vi "XMLPublishNode.vi"(8 "Error In":errorcluster, 9 "parent opcua path":string, 10 "OPC UA server refnum in":refnum<k21>, 11 "DOM node":refnum<k20>) -> (0 "Error Out":errorcluster, 2 "OPC UA server refnum out":refnum<k21>, 3 "DOM node (dup)":refnum<k20>)   [LabVIEW 2014, in "OPCUA XML.lvlib"]
uses:
  OPCUA XML.lvlib
  <vilib>/xml/Close Reference(Node).vi
  <vilib>/xml/Close Reference(NNMap).vi
  <resource>/objmgr/DOMUserDefRef.rc
  <vilib>/xml/NI_XML.lvlib
  <vilib>/OPCUA/NI OPC UA Server.lvlib
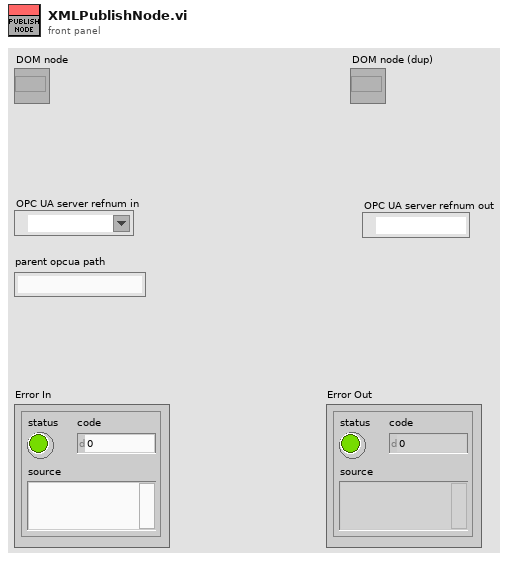
[diagram p1: front panel]
types:
  T1 = cluster{"name":string, "data type":u16, "access level":u16, "description":string}
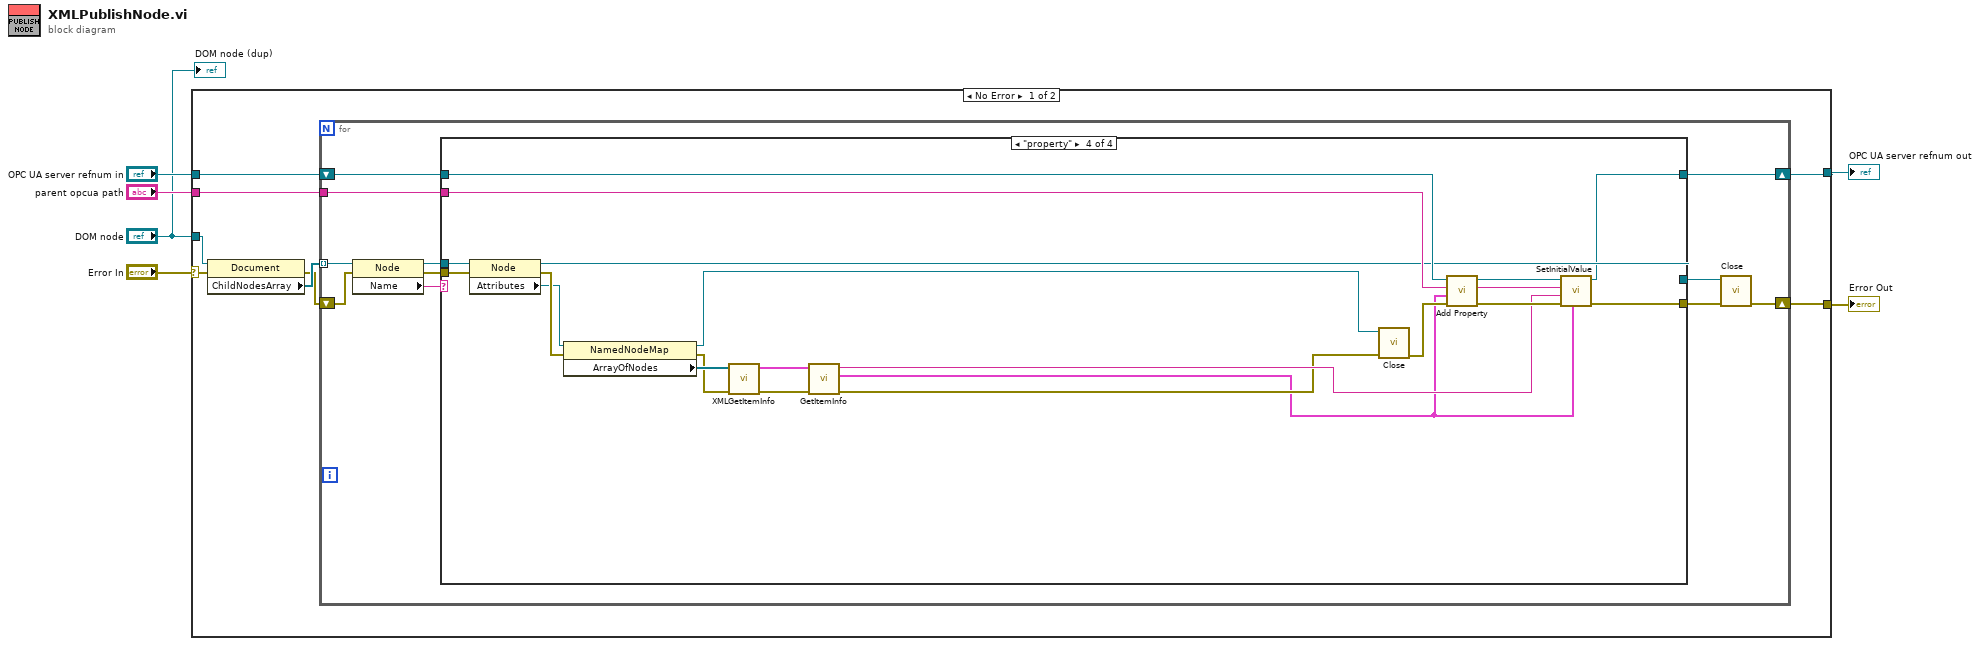
[diagram p0: block diagram]
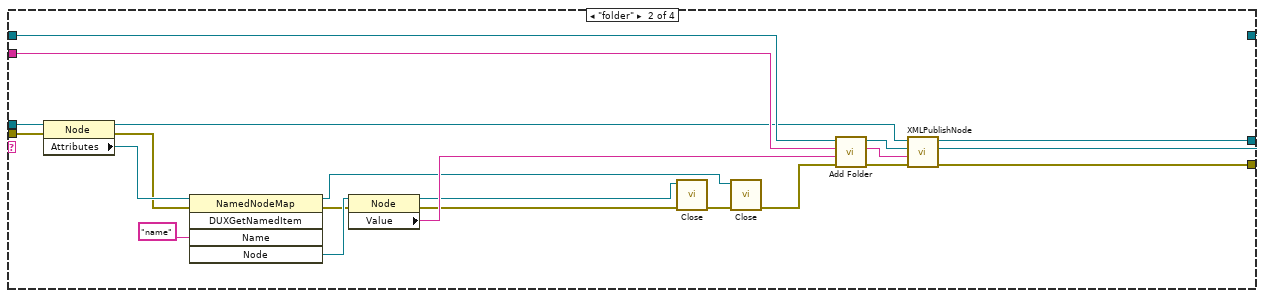
[diagram p3: hidden frame]
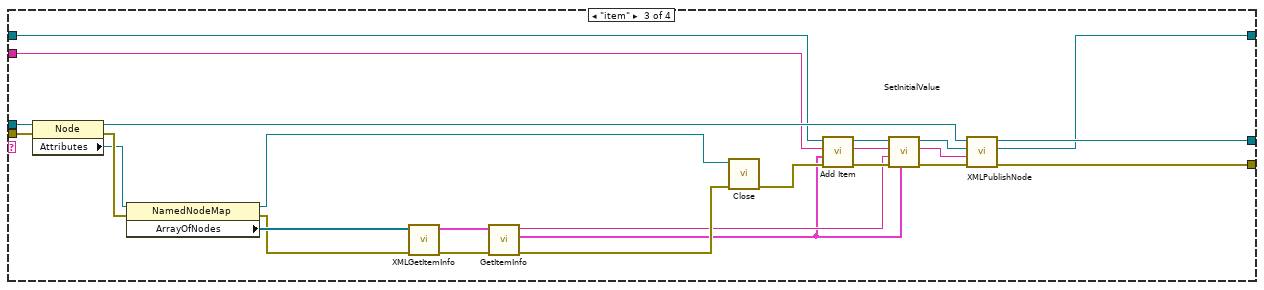
[diagram p4: hidden frame]
diagram:
  n1 = case shown="No Error" "Error In" {
    selector: "Error In" -> [w8 w98]
    tunnel: [w12 w98] -> w6
    tunnel: "DOM node" -> [w14 _]
    tunnel: "parent opcua path" -> [w11 _]
    tunnel: "OPC UA server refnum in" -> [w10 w97]
    tunnel: [w9 w97] -> w2
    frame No Error {
      n2 = property class="Document"(reference=w14, error in=w8) -> (error out=w7:errorcluster, "ChildNodesArray"=w13:refnum<k20>[])  [unwired: 1 out]
      n3 = for {
        tunnel: w13 -> [w25] mode=indexing
        shift-right: [w21] -> w12
        shift-left: w7 -> [w22]
        tunnel: w11 -> [w20]
        shift-right: [w18] -> w9
        shift-left: w10 -> [w19]
        n4 = property class="Node"(reference=w25, error in=w22) -> (reference out=w23:refnum<k20>, error out=w17:errorcluster, "Name"=w24:string)
        n5 = case shown="\"property\"" w24 {
          tunnel: w23 -> [w27 w50 w75 w91]
          tunnel: w20 -> [_ w46 w71 w95]
          tunnel: w19 -> [w26 w45 w72 w96]
          tunnel: [w26 w39 w70 w85] -> w18
          tunnel: w17 -> [w28 w36 w68 w90]
          tunnel: [w27 w42 w74 w89] -> w16
          tunnel: [w28 w41 w69 w84] -> w15
          frame Default {
          }
          frame "folder" {
            n6 = property class="Node"(reference=w50, error in=w36) -> (reference out=w43:refnum<k20>, error out=w35:errorcluster, "Attributes"=w49:refnum<k20>)
            n7 = invoke class="NamedNodeMap" method="DUXGetNamedItem"(reference=w49, error in=w35, "Name"="name") -> (reference out=w30:refnum<k20>, error out=w34:errorcluster, "Node"=w47:refnum<k20>)  [unwired: 2 in, 2 out]
            n8 = property class="Node"(reference=w47, error in=w34) -> (reference out=w29:refnum<k20>, error out=w33:errorcluster, "Value"=w44:string)
            n9 = call-poly <vilib>:"Close.vi"("error in (no error)"=w33, "node"=w29) -> ("error out"=w32:errorcluster)  [unwired: 7 out]
            n10 = call-poly <vilib>:"Close.vi"("error in (no error)"=w32, "named node map"=w30) -> ("error out"=w31:errorcluster)  [unwired: 7 out]
            n11 = call <vilib>:"Add Folder.vi"("error in (no error)"=w31, "folder name"=w44, "parent folder path"=w46, "OPC UA server refnum in"=w45) -> ("error out"=w37:errorcluster, "folder path"=w38:string, "OPC UA server refnum out"=w40:refnum<k21>)  [unwired: 4 in]
            n12 = call "XMLPublishNode.vi"("Error In"=w37, "parent opcua path"=w38, "OPC UA server refnum in"=w40, "DOM node"=w43) -> ("Error Out"=w41:errorcluster, "OPC UA server refnum out"=w39:refnum<k21>, "DOM node (dup)"=w42:refnum<k20>)  [unwired: 5 in]
          }
          frame "item" {
            n13 = property class="Node"(reference=w75, error in=w68) -> (reference out=w73:refnum<k20>, error out=w67:errorcluster, "Attributes"=w66:refnum<k20>)
            n14 = property class="NamedNodeMap"(reference=w66, error in=w67) -> (reference out=w65:refnum<k20>, error out=w56:errorcluster, "ArrayOfNodes"=w57:refnum<k20>[])
            n15 = call "XMLGetItemInfo.vi"("error in (no error)"=w56, "ArrayOfNodes"=w57) -> ("error out"=w55:errorcluster, "Array"=w54:cluster{"Name":string, "Value":string}[])  [unwired: 8 in]
            n16 = call "GetItemInfo.vi"("error in (no error)"=w55, "Array"=w54) -> ("error out"=w53:errorcluster, "item"=w51:T1, "Value"=w52:string)  [unwired: 7 in]
            n17 = call-poly <vilib>:"Close.vi"("error in (no error)"=w53, "named node map"=w65) -> ("error out"=w64:errorcluster)  [unwired: 7 out]
            n18 = call <vilib>:"Add Item.vi"("error in (no error)"=w64, "item"=w51, "parent folder path"=w71, "OPC UA server refnum in"=w72) -> ("error out"=w61:errorcluster, "item path"=w62:string, "OPC UA server refnum out"=w63:refnum<k21>)  [unwired: 4 in]
            n19 = call "SetInitialValue.vi"("item"=w51, "Error In"=w61, "value string"=w52, "node path"=w62, "OPC UA server refnum in"=w63) -> ("Error Out"=w60:errorcluster, "node path (dup)"=w58:string, "OPC UA server refnum out"=w59:refnum<k21>)  [unwired: 4 in]
            n20 = call "XMLPublishNode.vi"("Error In"=w60, "parent opcua path"=w58, "OPC UA server refnum in"=w59, "DOM node"=w73) -> ("Error Out"=w69:errorcluster, "OPC UA server refnum out"=w70:refnum<k21>, "DOM node (dup)"=w74:refnum<k20>)  [unwired: 5 in]
          }
          frame "property" {
            n21 = property class="Node"(reference=w91, error in=w90) -> (reference out=w89:refnum<k20>, error out=w94:errorcluster, "Attributes"=w93:refnum<k20>)
            n22 = property class="NamedNodeMap"(reference=w93, error in=w94) -> (reference out=w92:refnum<k20>, error out=w79:errorcluster, "ArrayOfNodes"=w80:refnum<k20>[])
            n23 = call "XMLGetItemInfo.vi"("error in (no error)"=w79, "ArrayOfNodes"=w80) -> ("error out"=w82:errorcluster, "Array"=w81:cluster{"Name":string, "Value":string}[])  [unwired: 8 in]
            n24 = call "GetItemInfo.vi"("error in (no error)"=w82, "Array"=w81) -> ("error out"=w77:errorcluster, "item"=w76:T1, "Value"=w78:string)  [unwired: 7 in]
            n25 = call-poly <vilib>:"Close.vi"("error in (no error)"=w77, "named node map"=w92) -> ("error out"=w88:errorcluster)  [unwired: 7 out]
            n26 = call <vilib>:"Add Property.vi"("error in (no error)"=w88, "property"=w76, "item path"=w95, "OPC UA server refnum in"=w96) -> ("error out"=w86:errorcluster, "property path"=w83:string, "OPC UA server refnum out"=w87:refnum<k21>)  [unwired: 4 in]
            n27 = call "SetInitialValue.vi"("item"=w76, "Error In"=w86, "value string"=w78, "node path"=w83, "OPC UA server refnum in"=w87) -> ("Error Out"=w84:errorcluster, "OPC UA server refnum out"=w85:refnum<k21>)  [unwired: 4 in, 1 out]
          }
        }
        n28 = call-poly <vilib>:"Close.vi"("error in (no error)"=w15, "node"=w16) -> ("error out"=w21:errorcluster)  [unwired: 7 out]
      }
    }
    frame Error {
    }
  }
  "Error Out" <- w6
  "OPC UA server refnum out" <- w2
  "DOM node (dup)" <- "DOM node"
